vi "Compare Class Type.vi"(4 "MusicElement Check":refnum<class "MusicElement.lvclass">, 5 "MusicElement in":refnum<class "MusicElement.lvclass">) -> (1 "Same Class Type?":bool)   [LabVIEW 2015, in "MusicElement.lvclass"]
uses:
  MusicElement.lvclass
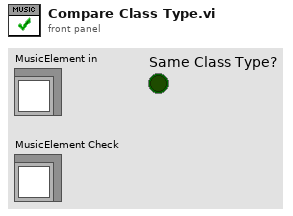
[diagram p1: front panel]
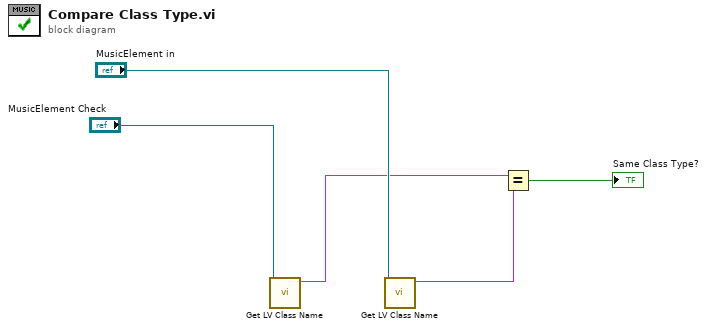
[diagram p0: block diagram]
diagram:
  n1 = call <vilib>:"Get LV Class Name.vi"("object"="MusicElement Check") -> ("class name"=w1:string)  [unwired: 9 in, 1 out]
  n2 = call <vilib>:"Get LV Class Name.vi"("object"="MusicElement in") -> ("class name"=w2:string)  [unwired: 9 in, 1 out]
  n3 = Equal?(x=w1, y=w2) -> (x = y?=→"Same Class Type?":bool)
